vi "PH_Cam_BaseClass.Proc Prc Prdc.vi"(0 "VI in":refnum<vi>, 2 "Image In":T1, 5 "error in (no error)":errorcluster) -> (14 "VI out":refnum<vi>, 19 "error out":errorcluster)   [LabVIEW 2014, in "PH_Cam_BaseClass.lvlib"]
uses:
  PH_Cam_BaseClass.lvlib
  <vilib>/vision/Image Controls.llb/IMAQ Image.ctl
  <vilib>/vision/NI_Vision_Development_Module.lvlib
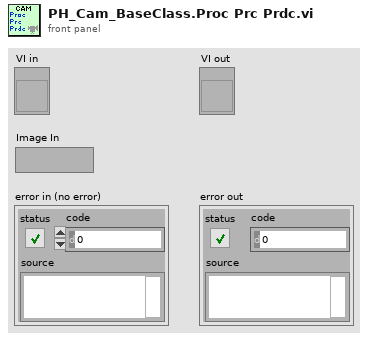
[diagram p1: front panel]
types:
  T1 = typedef "IMAQ Image.ctl" = refnum<image>
  T2 = typedef "PH_Cam_BaseClass.lvlib/PH_Cam_BaseClass.i attribute.ctl" = cluster{"Gui Refs":T3, "Cam":cluster{"Source Notifier":refnum<notifier>, "Error":errorcluster, "Camera ID":string}, "Images":cluster{"Cam":T1, "Operation":T1, "PSDB":T1}, "Window Image":cluster{"Indicate Image":bool, "Window No.":i32, "Scale Facor":dbl, "Center Cross":bool, "Subtract Backgr":bool, "CoG":bool, "Color Palette":cluster{"Red":u8, "Green":u8, "Blue":u8}[], "Image On":bool}, "Default Prdc Int":i32, "Performance":cluster{"on":bool, "Timestamp Last Frame":i32}, "Histogram":cluster{"on":bool, "Mapping":bool}, "Save Image":cluster{"Save":bool, "File refnum":refnum<file>}, "Setting Service ID":i32, "Screen":cluster{"x-resolution":i16, "y-resolution":i16}, "On":bool, "Constructor finished":bool, "configured":bool}
  T3 = typedef "PH_Cam_BaseClass.lvlib/PH_Cam_BaseClass.GUI Refs.ctl" = cluster{"Frame Rate":refnum<vi>, "Get Frame Rate":refnum<vi>, "Show Image":refnum<vi>, "Get Histogram":refnum<vi>, "Mapping":refnum<vi>, "Histogram":refnum<vi>, "Center Cross":refnum<vi>, "Center of Gravity":refnum<vi>, "Scale Factor [%]":refnum<vi>, "Save Image":refnum<vi>, "Palette":refnum<vi>, "Subtract Background":refnum<vi>, "Cam Error":refnum<vi>, "On":refnum<vi>, "Cam List":refnum<vi>}
  T4 = typedef "Image Type" = u32
  T5 = cluster{"Starting Value":sgl, "Incremental Value":sgl, "Histogram":u32[]}
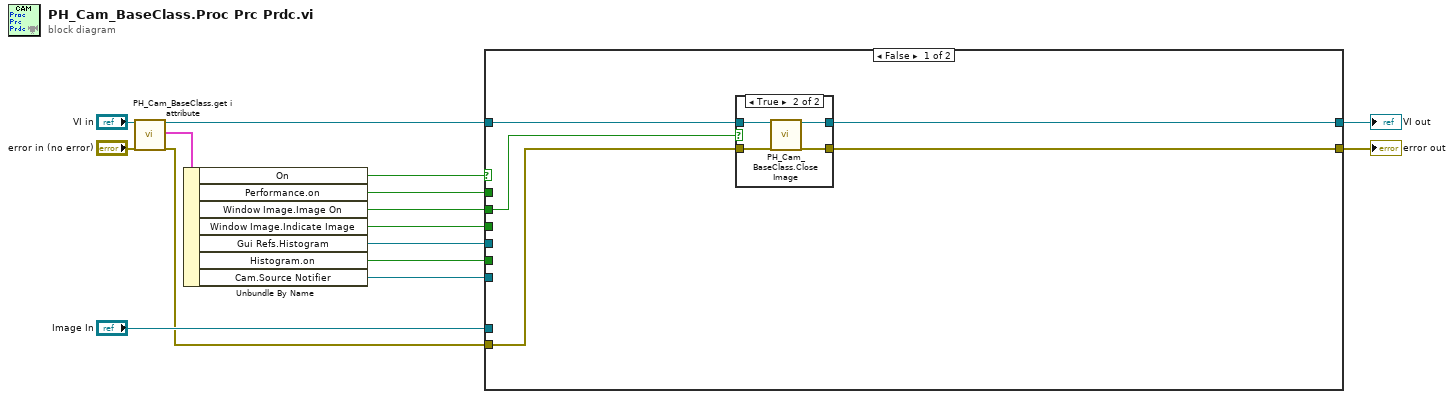
[diagram p0: block diagram]
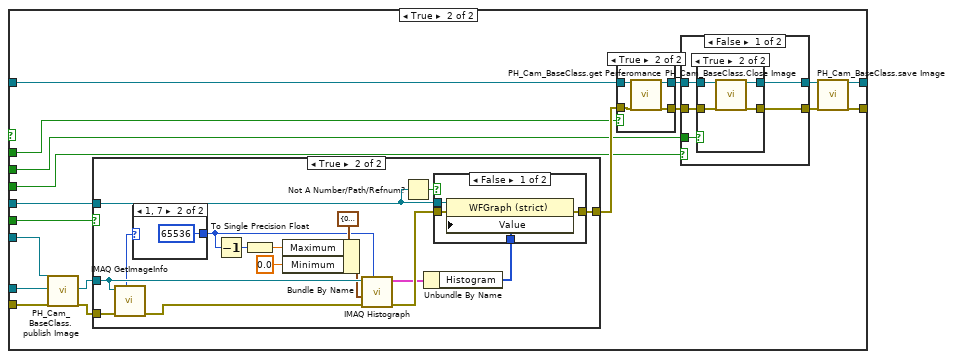
[diagram p3: hidden frame]
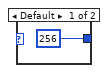
[diagram p6: hidden frame]
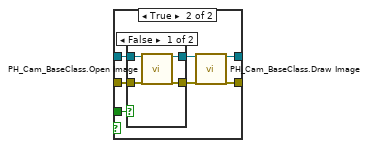
[diagram p9: hidden frame]
diagram:
  n1 = call "PH_Cam_BaseClass.get i attribute.vi"("i ref in"="VI in", "error in (no error)"="error in (no error)") -> ("i ref out"=w2:refnum<vi>, "i attribute"=w5:T2, "error out"=w11:errorcluster)  [unwired: 15 in]
  n2 = Unbundle By Name(w5) -> ("On"=w1:bool, "Performance.on"=w6:bool, "Window Image.Image On"=w12:bool, "Window Image.Indicate Image"=w7:bool, "Gui Refs.Histogram"=w8:refnum<vi>, "Histogram.on"=w9:bool, "Cam.Source Notifier"=w10:refnum<notifier>)
  n3 = case shown="False" w1 {
    tunnel: "Image In" -> [_ w44]
    tunnel: w12 -> [w16 w36]
    tunnel: w11 -> [w18 w35]
    tunnel: w10 -> [_ w34]
    tunnel: w9 -> [_ w33]
    tunnel: w8 -> [_ w32]
    tunnel: w7 -> [_ w31]
    tunnel: w6 -> [_ w30]
    tunnel: [w17 w29] -> w4
    tunnel: [w19 w28] -> w3
    tunnel: w2 -> [w20 w27]
    frame False {
      n4 = case shown="True" w16 {
        tunnel: w20 -> [w22 w26]
        tunnel: [w22 w25] -> w19
        tunnel: w18 -> [w21 w24]
        tunnel: [w21 w23] -> w17
        frame False {
        }
        frame True {
          n5 = call "PH_Cam_BaseClass.Close Image.vi"("i ref in"=w26, "error in"=w24) -> ("i ref out"=w25:refnum<vi>, "error out"=w23:errorcluster)  [unwired: 16 in]
        }
      }
    }
    frame True {
      n6 = call "PH_Cam_BaseClass.publish Image.vi"("Notifier"=w34, "Image In"=w44, "error in (no error)"=w35) -> ("Image Out"=w39:T1, "error out"=w41:errorcluster)  [unwired: 15 in]
      n7 = case shown="True" w33 {
        tunnel: w41 -> [w51 w60]
        tunnel: w39 -> [_ w61]
        tunnel: [w51 w66] -> w42
        tunnel: w32 -> [_ w62]
        frame False {
        }
        frame True {
          n8 = call "IMAQ GetImageInfo"("error in (no error)"=w60, "Image"=w61) -> ("error out"=w59:errorcluster, "Image Type"=w58:T4)  [unwired: 2 in, 6 out]
          n9 = case shown="1, 7" w58 {
            tunnel: [256 ("Number of Classes") 65536 ("Number of Classes")] -> w55
            frame Default {
            }
            frame 1, 7 {
            }
          }
          n10 = Decrement(x=w55) -> (x-1=w54:i32)
          n11 = To Single Precision Float(number=w54) -> (single precision float=w53:sgl)
          n12 = Bundle By Name(cluster=cluster{"Minimum":sgl, "Maximum":sgl} {"Minimum"=0.0, "Maximum"=0.0} ("output cluster"), "Maximum"=w53, "Minimum"=sgl 0.0) -> (w57:cluster{"Minimum":sgl, "Maximum":sgl})
          n13 = call "IMAQ Histograph"("Number of Classes"=w55, "error in (no error)"=w59, "Interval Range"=w57, "Image"=w61) -> ("error out"=w67:errorcluster, "Histogram Graph"=w64:T5)  [unwired: 4 in, 2 out]
          n14 = Not A Number/Path/Refnum?(number/path/refnum=w62) -> (NaN/Path/Refnum?=w65:bool)
          n15 = Unbundle By Name(w64) -> ("Histogram"=w63:u32[])
          n16 = case shown="False" w65 {
            tunnel: w67 -> [w73 w74]
            tunnel: [w72 w74] -> w66
            tunnel: w62 -> [w71 _]
            tunnel: w63 -> [w70 _]
            frame False {
              n17 = property class="WFGraph (strict)"(reference=w71, error in=w73, "Value"=w70) -> (error out=w72:errorcluster)  [unwired: 1 out]
            }
            frame True {
            }
          }
        }
      }
      n18 = case shown="True" w30 {
        tunnel: w27 -> [w46 w50]
        tunnel: [w46 w49] -> w37
        tunnel: w42 -> [w45 w48]
        tunnel: [w45 w47] -> w38
        frame False {
        }
        frame True {
          n19 = call "PH_Cam_BaseClass.get Perferomance.vi"("i ref in"=w50, "error in (no error)"=w48) -> ("i ref out"=w49:refnum<vi>, "error out"=w47:errorcluster)  [unwired: 16 in]
        }
      }
      n20 = case shown="False" w31 {
        tunnel: w38 -> [w79 w88]
        tunnel: [w78 w92] -> w43
        tunnel: w37 -> [w77 w90]
        tunnel: [w76 w91] -> w40
        tunnel: w36 -> [w75 w86]
        frame False {
          n21 = case shown="True" w75 {
            tunnel: w79 -> [w80 w85]
            tunnel: [w80 w84] -> w78
            tunnel: w77 -> [w81 w83]
            tunnel: [w81 w82] -> w76
            frame False {
            }
            frame True {
              n22 = call "PH_Cam_BaseClass.Close Image.vi"("i ref in"=w83, "error in"=w85) -> ("i ref out"=w82:refnum<vi>, "error out"=w84:errorcluster)  [unwired: 16 in]
            }
          }
        }
        frame True {
          n23 = case shown="False" w86 {
            tunnel: w90 -> [w96 w98]
            tunnel: [w95 w98] -> w89
            tunnel: w88 -> [w94 w97]
            tunnel: [w93 w97] -> w87
            frame False {
              n24 = call "PH_Cam_BaseClass.Open Image.vi"("i ref in"=w96, "error in"=w94) -> ("i ref out"=w95:refnum<vi>, "error out"=w93:errorcluster)  [unwired: 16 in]
            }
            frame True {
            }
          }
          n25 = call "PH_Cam_BaseClass.Draw Image.vi"("i ref in"=w89, "error in (no error)"=w87) -> ("i ref out"=w91:refnum<vi>, "error out"=w92:errorcluster)  [unwired: 16 in]
        }
      }
      n26 = call "PH_Cam_BaseClass.save Image.vi"("i ref in"=w40, "error in (no error)"=w43) -> ("i ref out"=w28:refnum<vi>, "error out"=w29:errorcluster)  [unwired: 16 in]
    }
  }
  "error out" <- w4
  "VI out" <- w3
